vi "Flash.vi"(8 "Flash Position":cluster{"X":i32, "Y":i32}, 11 "Grid In":i64[][](array[numeric])) -> (0 "New Flashes":cluster{"X":i32, "Y":i32}[](array[cluster]), 3 "Grid Out":i64[][](array[numeric]))   [LabVIEW 2021]
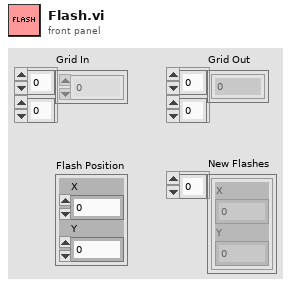
[diagram p1: front panel]
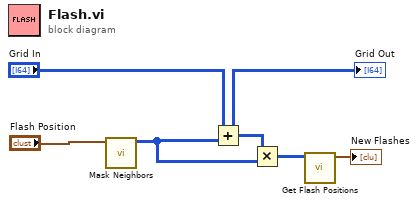
[diagram p0: block diagram]
diagram:
  n1 = call "Mask Neighbors.vi"("Flash Position"="Flash Position") -> ("Neigbor Mask"=w1:i64[][])  [unwired: 10 in]
  n2 = Add(x="Grid In", y=w1) -> (x+y=w6:i64[][])
  "Grid Out" <- w6
  n3 = Multiply(x=w6, y=w1) -> (x*y=w5:i64[][])
  n4 = call "Get Flash Positions.vi"("Grid In"=w5) -> ("Flash Positions"=→"New Flashes":cluster{"X":i32, "Y":i32}[])  [unwired: 10 in]
